vi "data parsing(debug2).vi"(11 "배열":string[](array[string])) -> (1 "Filtered Sensor":u32[][](array[numeric]), 2 "No Filter Sensor":u32[][](array[numeric]), 3 "Time":string[](array[string]))   [LabVIEW 2015]
panel:
  out "Filtered Sensor 6":u32[](array[numeric])
  out "Filtered Sensor 5":u32[](array[numeric])
  out "Filtered Sensor 4":u32[](array[numeric])
  out "Filtered Sensor 3":u32[](array[numeric])
  out "Filtered Sensor 2":u32[](array[numeric])
  out "Filtered Sensor 1":u32[](array[numeric])
  out "No Filter Sensor 6":u32[](array[numeric])
  out "No Filter Sensor 5":u32[](array[numeric])
  out "No Filter Sensor 4":u32[](array[numeric])
  out "No Filter Sensor 3":u32[](array[numeric])
  out "No Filter Sensor 2":u32[](array[numeric])
  out "No Filter Sensor 1":u32[](array[numeric])
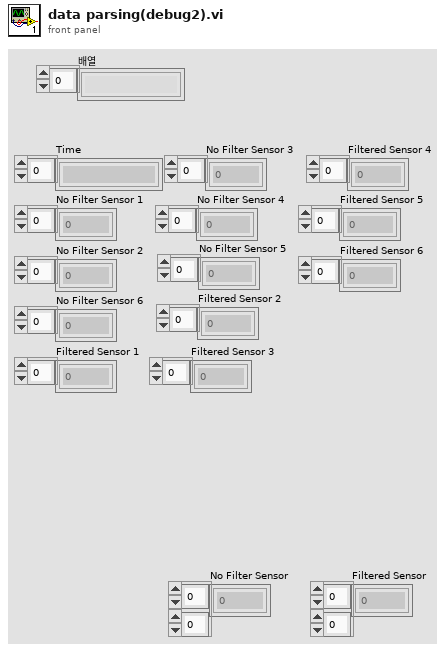
[diagram p1: front panel]
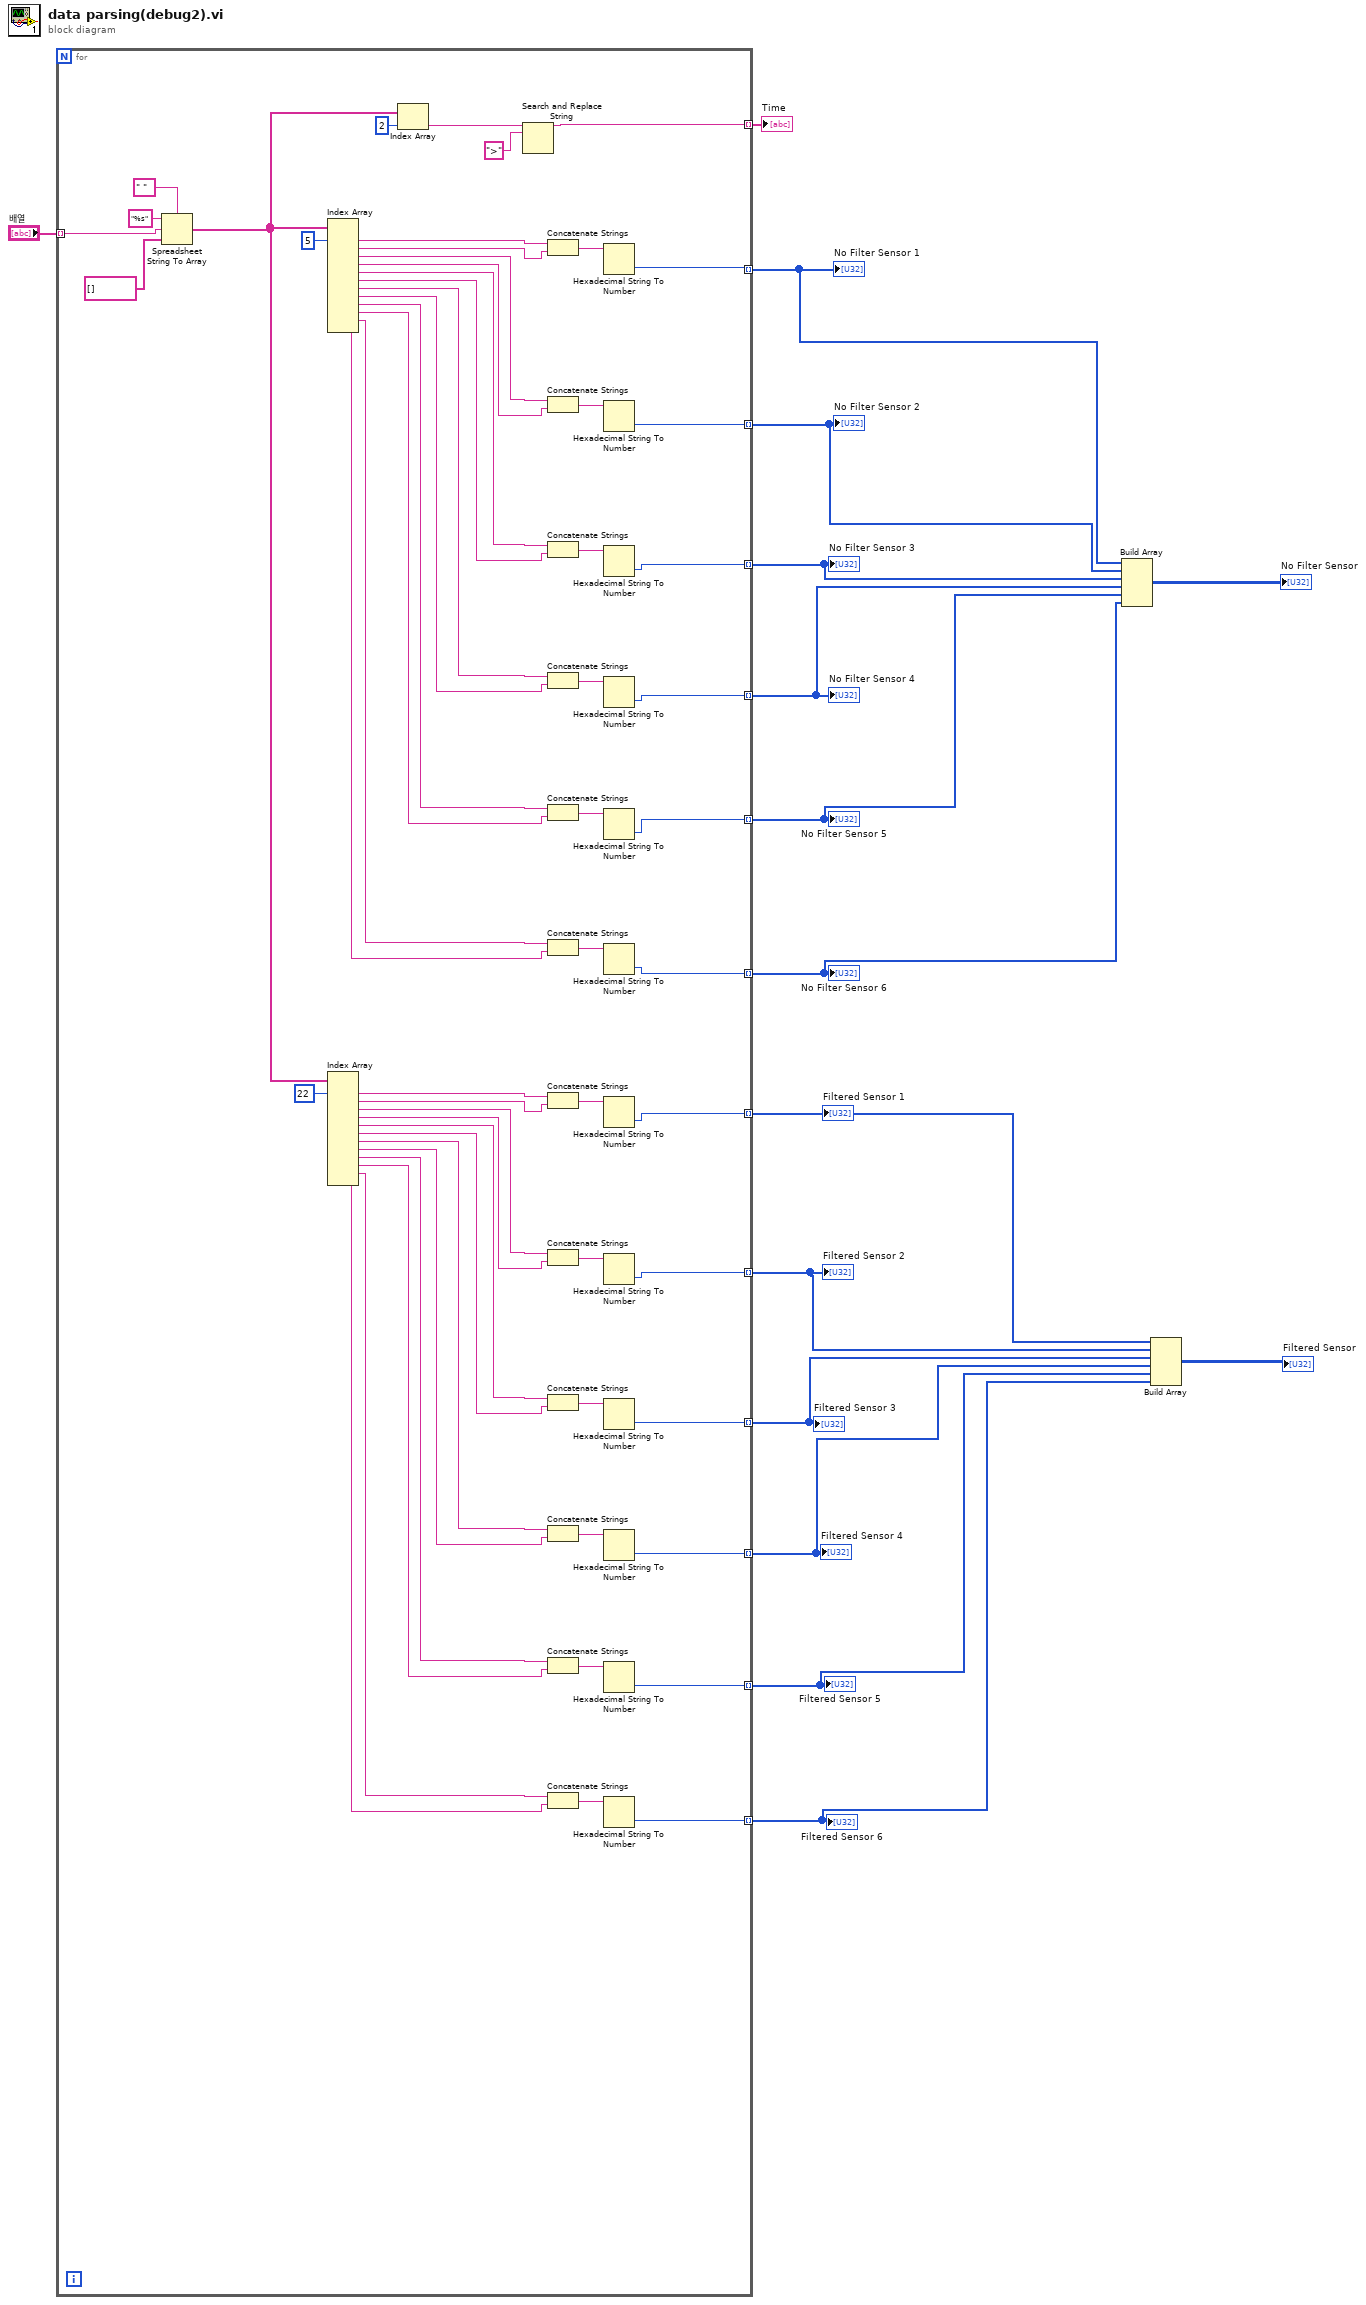
[diagram p0: block diagram]
diagram:
  n1 = for {
    tunnel: "배열" -> [w62] mode=indexing
    tunnel: [w41] -> w15 mode=indexing
    tunnel: [w28] -> w12 mode=indexing
    tunnel: [w27] -> w13 mode=indexing
    tunnel: [w26] -> w14 mode=indexing
    tunnel: [w25] -> w11 mode=indexing
    tunnel: [w24] -> w10 mode=indexing
    tunnel: [w23] -> w9 mode=indexing
    tunnel: [w22] -> w6 mode=indexing
    tunnel: [w21] -> w5 mode=indexing
    tunnel: [w20] -> w4 mode=indexing
    tunnel: [w19] -> w3 mode=indexing
    tunnel: [w18] -> w2 mode=indexing
    tunnel: [w17] -> w1 mode=indexing
    n2 = Spreadsheet String To Array(delimiter (Tab)=" " ("구분 문자(탭)"), format string="%s" ("포맷 문자열"), spreadsheet string=w62, array type (2D Dbl)=string[] []) -> (array=w43:string[])
    n3 = Index Array(array=w43, index #1=5 ("비활성화된 인덱스 (열)")) -> (element #1=w75:string, element #2=w74:string, element #3=w73:string, element #4=w72:string, element #5=w71:string, element #6=w70:string, element #7=w69:string, element #8=w68:string, element #9=w67:string, element #10=w66:string, element #11=w58:string, element #12=w57:string)  [unwired: 11 in]
    n4 = Index Array(array=w43, index #1=22 ("비활성화된 인덱스 (열)")) -> (element #1=w44:string, element #2=w45:string, element #3=w46:string, element #4=w47:string, element #5=w48:string, element #6=w49:string, element #7=w50:string, element #8=w51:string, element #9=w52:string, element #10=w53:string, element #11=w55:string, element #12=w56:string)  [unwired: 11 in]
    n5 = Index Array(array=w43, index=2 ("비활성화된 인덱스 (열)")) -> (element=w65:string)
    n6 = Search and Replace String(input string=w65, search string=">" ("검색 문자열")) -> (result string=w41:string)  [unwired: 6 in, 3 out]
    n7 = Concatenate Strings(w75, w74) -> (w40:string)
    n8 = Concatenate Strings(w73, w72) -> (w39:string)
    n9 = Concatenate Strings(w71, w70) -> (w38:string)
    n10 = Concatenate Strings(w69, w68) -> (w37:string)
    n11 = Concatenate Strings(w67, w66) -> (w36:string)
    n12 = Concatenate Strings(w58, w57) -> (w35:string)
    n13 = Concatenate Strings(w44, w45) -> (w34:string)
    n14 = Concatenate Strings(w46, w47) -> (w32:string)
    n15 = Concatenate Strings(w48, w49) -> (w33:string)
    n16 = Concatenate Strings(w50, w51) -> (w31:string)
    n17 = Concatenate Strings(w52, w53) -> (w30:string)
    n18 = Concatenate Strings(w55, w56) -> (w29:string)
    n19 = Hexadecimal String To Number(string=w40) -> (number=w28:u32)  [unwired: 2 in, 1 out]
    n20 = Hexadecimal String To Number(string=w39) -> (number=w27:u32)  [unwired: 2 in, 1 out]
    n21 = Hexadecimal String To Number(string=w38) -> (number=w26:u32)  [unwired: 2 in, 1 out]
    n22 = Hexadecimal String To Number(string=w37) -> (number=w25:u32)  [unwired: 2 in, 1 out]
    n23 = Hexadecimal String To Number(string=w36) -> (number=w24:u32)  [unwired: 2 in, 1 out]
    n24 = Hexadecimal String To Number(string=w35) -> (number=w23:u32)  [unwired: 2 in, 1 out]
    n25 = Hexadecimal String To Number(string=w34) -> (number=w22:u32)  [unwired: 2 in, 1 out]
    n26 = Hexadecimal String To Number(string=w32) -> (number=w21:u32)  [unwired: 2 in, 1 out]
    n27 = Hexadecimal String To Number(string=w33) -> (number=w20:u32)  [unwired: 2 in, 1 out]
    n28 = Hexadecimal String To Number(string=w31) -> (number=w19:u32)  [unwired: 2 in, 1 out]
    n29 = Hexadecimal String To Number(string=w30) -> (number=w18:u32)  [unwired: 2 in, 1 out]
    n30 = Hexadecimal String To Number(string=w29) -> (number=w17:u32)  [unwired: 2 in, 1 out]
  }
  "Time" <- w15
  "No Filter Sensor 1" <- w12
  "No Filter Sensor 2" <- w13
  "No Filter Sensor 3" <- w14
  "No Filter Sensor 4" <- w11
  "No Filter Sensor 5" <- w10
  "No Filter Sensor 6" <- w9
  "Filtered Sensor 1" <- w6
  "Filtered Sensor 2" <- w5
  "Filtered Sensor 3" <- w4
  "Filtered Sensor 4" <- w3
  "Filtered Sensor 5" <- w2
  "Filtered Sensor 6" <- w1
  n31 = Build Array(w12, w13, w14, w11, w10, w9) -> (→"No Filter Sensor":u32[][])
  n32 = Build Array(w6, w5, w4, w3, w2, w1) -> (→"Filtered Sensor":u32[][])
